vi "parse tag header.vi"(8 "error in":errorcluster, 10 "tag type name":string="dataTag", 11 "Path":path) -> (0 "error out":errorcluster, 1 "classifications":T1[](array[typedef]), 2 "types":T2[](array[typedef]), 3 "names":string[](array[string]))   [LabVIEW 2013, in "Shared Library Module configuration.lvclass"]
uses:
  Shared Library Module configuration.lvclass
  <vilib>/NI/Tag Bus/tag/Data Type.ctl
  <vilib>/NI/Tag Bus Module Framework/channel/channel classification.ctl
  <vilib>/NI/Tag Bus/tag/tag descriptor.lvclass
  <vilib>/NI/Tag Bus Module Framework/channel/TBM channel.lvclass
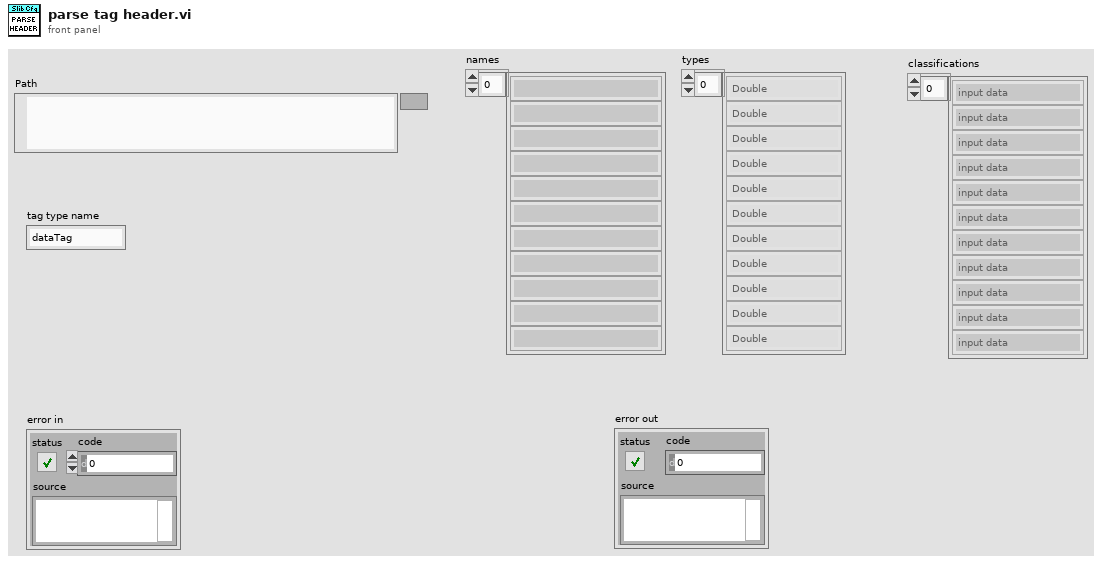
[diagram p1: front panel]
types:
  T1 = typedef "TBM channel.lvclass/channel classification.ctl" = enum16{"input data", "output data", "processing parameter", "processing result"}
  T2 = typedef "tag bus.lvlib/tag descriptor.lvclass/Data Type.ctl" = enum16{"Double", "Single", "I64", "I32", "I16", "I8", "U64", "U32", "U16", "U8", "Boolean", "String", "Array of Double", "Array of Single", "Array of I64", "Array of I32", "Array of I16", "Array of I8", "Array of U64", "Array of U32", "Array of U16", "Array of U8", "Array of Boolean", "Array of String"}
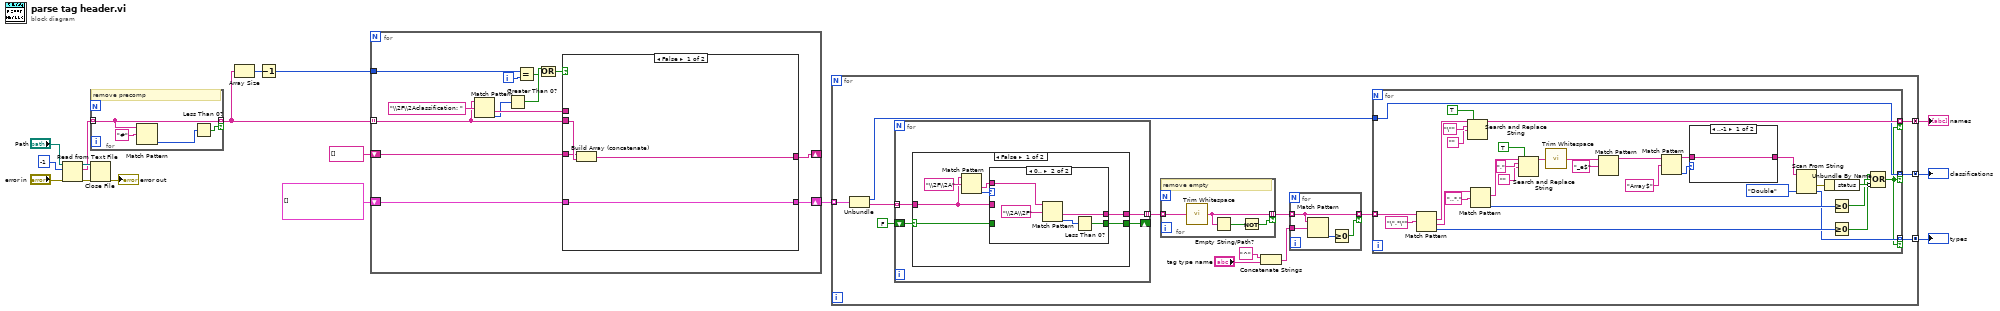
[diagram p0: block diagram]
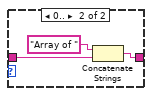
[diagram p2: hidden frame]
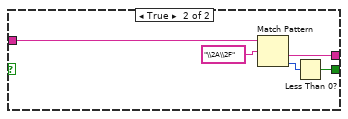
[diagram p4: hidden frame]
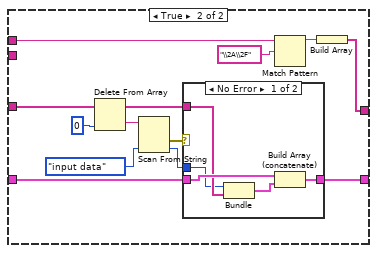
[diagram p5: hidden frame]
diagram:
  n1 = Read from Text File(file (use dialog)="Path", count=-1, error in="error in") -> (refnum out=w13:refnum<file>, text=w11:string[], error out=w12:errorcluster)  [unwired: 1 in, 1 out]
  n2 = for {
    tunnel: w11 -> [w19] mode=indexing
    tunnel: [w19] -> w5 mode=indexing if=w17
    # "remove precomp"
    n3 = Match Pattern(string=w19, regular expression="#") -> (offset past match=w18:i32)  [unwired: 1 in, 3 out]
    n4 = Less Than 0?(x=w18) -> (x < 0?=w17:bool)
  }
  n5 = Close File(refnum=w13, error in=w12) -> (error out=→"error out":errorcluster)  [unwired: 1 out]
  n6 = Array Size(array=w5) -> (size(s)=w4:i32)
  n7 = Decrement(x=w4) -> (x-1=w3:i32)
  n8 = for {
    tunnel: w5 -> [w32] mode=indexing
    shift-right: [w31] -> _
    shift-left: string[] [] -> [w30]
    shift-right: [w29] -> w2
    shift-left: cluster{"channel classification":T1, string[]}[] [] -> [w28]
    tunnel: w3 -> [w24]
    i -> [w23]
    n9 = Match Pattern(string=w32, regular expression="\\2F\\2Aclassification: ") -> (after substring=w27:string, offset past match=w26:i32)  [unwired: 1 in, 2 out]
    n10 = Greater Than 0?(x=w26) -> (x > 0?=w25:bool)
    n11 = Equal?(x=w24, y=w23) -> (x = y?=w22:bool)
    n12 = Or(x=w25, y=w22) -> (x .or. y?=w21:bool)
    n13 = case shown="False" w21 {
      tunnel: w32 -> [w37 _]
      tunnel: [w36 w45] -> w31
      tunnel: w30 -> [w35 w44]
      tunnel: [w34 w50] -> w29
      tunnel: w28 -> [w34 w49]
      tunnel: w27 -> [_ w48]
      frame False {
        n14 = Build Array (concatenate)(w35, w37) -> (w36:string[])
      }
      frame True {
        n15 = Delete From Array(array=w44, index=0) -> (deleted portion=w41:string, array with subset deleted=w42:string[])  [unwired: 1 in]
        n16 = Scan From String(input string=w41, default 1=channel_classification."input data" ("channel classification")) -> (error out=w40:errorcluster, output 1=w38:T1)  [unwired: 3 in, 2 out]
        n17 = case shown="No Error" w40 {
          tunnel: [w54 w56] -> w50
          tunnel: w49 -> [w53 w56]
          tunnel: w42 -> [w52 _]
          tunnel: w38 -> [w51 _]
          frame No Error {
            n18 = Bundle("channel classification"=w51, w52) -> (w55:cluster{"channel classification":T1, string[]})  [unwired: 1 in]
            n19 = Build Array (concatenate)(w53, w55) -> (w54:cluster{"channel classification":T1, string[]}[])
          }
          frame Error {
          }
        }
        n20 = Match Pattern(string=w48, regular expression="\\2A\\2F") -> (before substring=w46:string)  [unwired: 1 in, 3 out]
        n21 = Build Array(w46) -> (w45:string[])
      }
    }
  }
  n22 = for {
    tunnel: [w62] -> w9 mode=concatenating
    tunnel: [w61] -> w8 mode=concatenating
    tunnel: w2 -> [w60] mode=indexing
    tunnel: [w57] -> w1 mode=concatenating
    n23 = Unbundle(w60) -> ("channel classification"=w58:T1, w59:string[])
    n24 = for {
      tunnel: w59 -> [w112] mode=indexing
      shift-right: [w110] -> _
      shift-left: FALSE -> [w111]
      tunnel: [w109] -> w66 mode=indexing
      n25 = case shown="False" w111 {
        selector: w111 -> [w114 _]
        tunnel: w112 -> [w113 w131]
        tunnel: [w116 w129] -> w110
        tunnel: [w115 w128] -> w109
        frame False {
          n26 = Match Pattern(string=w113, regular expression="\\2F\\2A") -> (after substring=w117:string, offset past match=w118:i32)  [unwired: 1 in, 2 out]
          n27 = case shown="0.." w118 {
            tunnel: w117 -> [_ w125]
            tunnel: [w121 w123] -> w116
            tunnel: [w120 w124] -> w115
            tunnel: w114 -> [w121 _]
            tunnel: w113 -> [w120 _]
            frame ..-1 {
            }
            frame 0.. {
              n28 = Match Pattern(string=w125, regular expression="\\2A\\2F") -> (after substring=w124:string, offset past match=w122:i32)  [unwired: 1 in, 2 out]
              n29 = Less Than 0?(x=w122) -> (x < 0?=w123:bool)
            }
          }
        }
        frame True {
          n30 = Match Pattern(string=w131, regular expression="\\2A\\2F") -> (after substring=w128:string, offset past match=w130:i32)  [unwired: 1 in, 2 out]
          n31 = Less Than 0?(x=w130) -> (x < 0?=w129:bool)
        }
      }
    }
    n32 = for {
      tunnel: [w133] -> w65 mode=indexing if=w134
      tunnel: w66 -> [w132] mode=indexing
      # "remove empty"
      n33 = call <vilib>:"Trim Whitespace.vi"("string"=w132) -> ("trimmed string"=w133:string)  [unwired: 1 in]
      n34 = Empty String/Path?(string/path=w133) -> (empty?=w135:bool)
      n35 = Not(x=w135) -> (.not. x?=w134:bool)
    }
    n36 = Concatenate Strings("^" ("string"), "tag type name") -> (w64:string)
    n37 = for {
      tunnel: w64 -> [w108]
      tunnel: w65 -> [w106] mode=indexing
      tunnel: [w106] -> w63 mode=indexing if=w105
      n38 = Match Pattern(string=w106, regular expression=w108) -> (offset past match=w107:i32)  [unwired: 1 in, 3 out]
      n39 = Greater Or Equal To 0?(x=w107) -> (x >= 0?=w105:bool)
    }
    n40 = for {
      tunnel: w63 -> [w100] mode=indexing
      tunnel: [w83] -> w61 mode=indexing if=w70
      tunnel: [w82] -> w62 mode=indexing if=w70
      tunnel: w58 -> [w71]
      tunnel: [w71] -> w57 mode=indexing if=w70
      n41 = Match Pattern(string=w100, regular expression="\".*\"") -> (match substring=w86:string, after substring=w98:string, offset past match=w96:i32)  [unwired: 1 in, 1 out]
      n42 = Search and Replace String(replace all?=TRUE ("replace all? (F)"), input string=w86, search string="\"", replace string="") -> (result string=w83:string)  [unwired: 4 in, 3 out]
      n43 = Match Pattern(string=w98, regular expression=",.*,") -> (match substring=w91:string, offset past match=w95:i32)  [unwired: 1 in, 2 out]
      n44 = Search and Replace String(replace all?=TRUE ("replace all? (F)"), input string=w91, search string=",", replace string="") -> (result string=w81:string)  [unwired: 4 in, 3 out]
      n45 = call <vilib>:"Trim Whitespace.vi"("string"=w81) -> ("trimmed string"=w80:string)  [unwired: 1 in]
      n46 = Match Pattern(string=w80, regular expression="_e$") -> (before substring=w78:string)  [unwired: 1 in, 3 out]
      n47 = Match Pattern(string=w78, regular expression="Array$") -> (before substring=w72:string, offset past match=w74:i32)  [unwired: 1 in, 2 out]
      n48 = case shown="..-1" w74 {
        tunnel: [w101 w103] -> w73
        tunnel: w72 -> [w101 w104]
        frame ..-1 {
        }
        frame 0.. {
          n49 = Concatenate Strings("Array of " ("string"), w104) -> (w103:string)
        }
      }
      n50 = Scan From String(input string=w73, default 1=Data_Type."Double" ("data type")) -> (error out=w76:errorcluster, output 1=w82:T2)  [unwired: 3 in, 2 out]
      n51 = Unbundle By Name(w76) -> ("status"=w94:bool)
      n52 = Greater Or Equal To 0?(x=w95) -> (x >= 0?=w93:bool)
      n53 = Greater Or Equal To 0?(x=w96) -> (x >= 0?=w92:bool)
      n54 = Compound Arithmetic op=OR(w92, w93, invert w94) -> (w70:bool)
    }
  }
  "names" <- w8
  "types" <- w9
  "classifications" <- w1
